vi "twitterSkipRemainingPhases.vi"(8 "error in":errorcluster, 9 "Prev Exp":T1(ring)=enum."Single Manip Jump", 10 "cell stats":T2={"Ihold (pA)"=-1000.0, "Rm (MOhms)"=0.0, "Ra (MOhms)"=0.0, "Cm (pF)"=0.0, "tau (ms)"=0.0, "Rt (MOhms)"=30.0, "Variance"=0.0, "STD"=0.0} {"STD" format="%010.2f"; "Variance" format="%010.2f"; "Rt (MOhms)" format="%010.2f"; "tau (ms)" format="%08.2g"; "Cm (pF)" format="%08.2f"; "Ra (MOhms)" format="%010.2f"; "Rm (MOhms)" format="%010.2f"; "Ihold (pA)" format="%010.2f"}, 11 "Prev Phase":string="B") -> (0 "error out":errorcluster, 2 "Skip Remaining":bool)   [LabVIEW 2019]
uses:
  <vilib>/LVH/i3 Twitter/Controls/Tweet.ctl
  wc_protocol_v1.003 Folder/whole_cell_protocol/Controls/cell_stats-v02.ctl
  <vilib>/LVH/i3 Twitter/i3-twitter.lvlib
panel:
  out "tweet sent":string
  in  "Continue Button":bool
  in  "Terminate Button":bool
  out "light on":bool
  out "New Tweets Read":T3[](array[typedef])
  # "The Cell/Patch looks to be comprimised, respond via twitter or the panel to proceed"
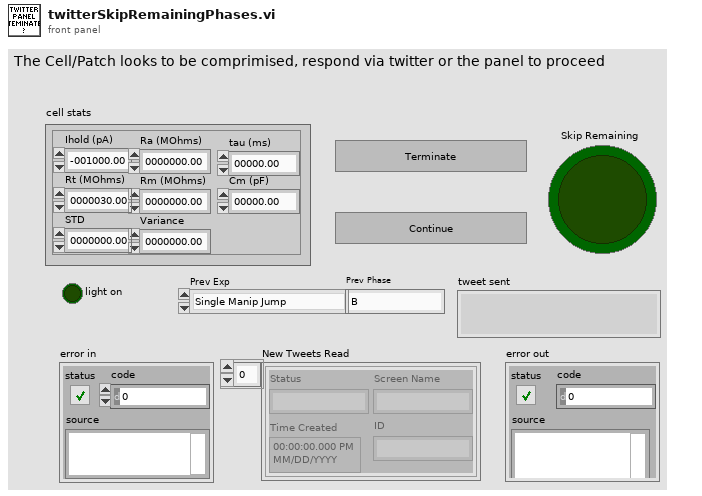
[diagram p1: front panel]
types:
  T1 = enum32{"Single Jump", "Solution Change", "Voltage Step", "Voltage Ramp", "Voltage Pulse", "Jump Train", "Paired Pulse", "Single Manip Jump", "Gap Free", "Multi M. Jump", "Current Pulse", "Current Ramp", "Gap Free Iclamp"}
  T2 = typedef "cell_stats-v02.ctl" = cluster{"Ihold (pA)":dbl, "Rm (MOhms)":dbl, "Ra (MOhms)":dbl, "Cm (pF)":dbl, "tau (ms)":dbl, "Rt (MOhms)":dbl, "Variance":dbl, "STD":dbl}
  T3 = typedef "i3-twitter.lvlib/Tweet.ctl" = cluster{"Status":string, "Time Created":timestamp, "Screen Name":string, "ID":string}
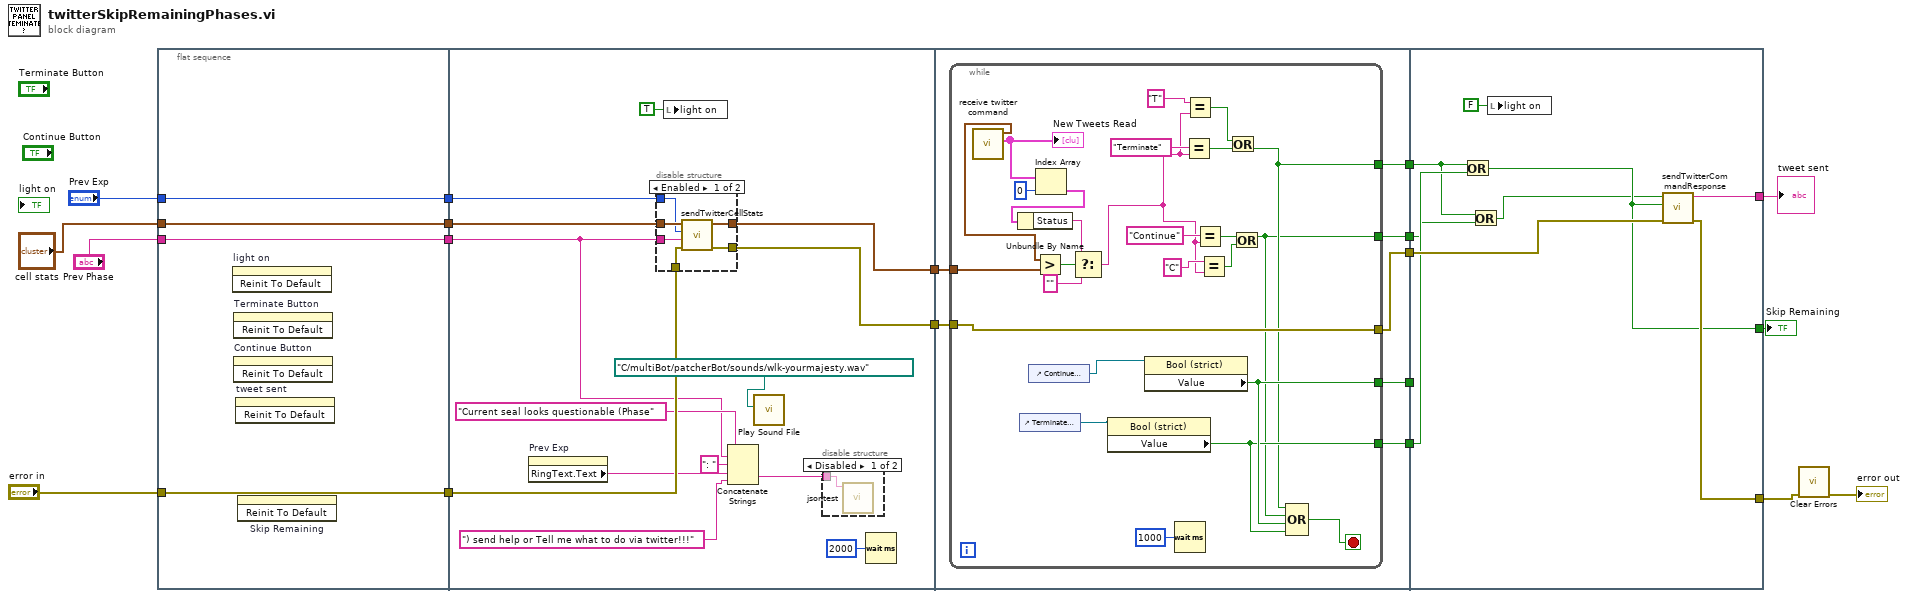
[diagram p0: block diagram]
diagram:
  n1 = flat-sequence {
    tunnel: "Prev Phase" -> [w20]
    tunnel: "Prev Exp" -> [w21]
    tunnel: "cell stats" -> [w22]
    tunnel: "error in" -> [w23]
    tunnel: [w23] -> w5
    tunnel: [w22] -> w4
    tunnel: [w21] -> w3
    tunnel: [w20] -> w2
    tunnel: [w35] -> w18
    tunnel: [w32] -> w7
    tunnel: w5 -> [w36]
    tunnel: w4 -> [w34]
    tunnel: w3 -> [w33]
    tunnel: w2 -> [w26]
    tunnel: w18 -> [w51]
    tunnel: [w50] -> w17
    tunnel: [w49] -> w15
    tunnel: [w48] -> w14
    tunnel: [w47] -> w13
    tunnel: [w46] -> w12
    tunnel: w7 -> [w45]
    tunnel: [w82] -> w19
    tunnel: w17 -> [w85]
    tunnel: [w84] -> w16
    tunnel: w15 -> [w80]
    tunnel: w14 -> [w81]
    tunnel: w13 -> [_]
    tunnel: w12 -> [w83]
    tunnel: [w78] -> w8
    frame #0 {
      n2 = invoke on="light on" class="Bool (strict)" method="Reinit To Default"() -> ()  [unwired: 3 in, 3 out]
      n3 = invoke on="Terminate Button" class="Bool (strict)" method="Reinit To Default"() -> ()  [unwired: 3 in, 3 out]
      n4 = invoke on="Continue Button" class="Bool (strict)" method="Reinit To Default"() -> ()  [unwired: 3 in, 3 out]
      n5 = invoke on="tweet sent" class="Str" method="Reinit To Default"() -> ()  [unwired: 3 in, 3 out]
      n6 = invoke on="Skip Remaining" class="Bool (strict)" method="Reinit To Default"() -> ()  [unwired: 3 in, 3 out]
    }
    frame #1 {
      n7 = property on="Prev Exp" class="Enum (strict)"() -> ("RingText.Text"=w25:string)  [unwired: 2 in, 2 out]
      n8 = disable-structure shown="Enabled" {
        disable-tunnel: w36 -> [w44 _]
        disable-tunnel: [w43 _] -> w35
        disable-tunnel: w34 -> [w42 _]
        disable-tunnel: w33 -> [w41 _]
        disable-tunnel: [w40 _] -> w32
        disable-tunnel: w26 -> [w39 _]
        frame Enabled {
          n9 = call "sendTwitterCellStats.vi"("error in"=w44, "Prev Phase"=w39, "Prev Exp"=w41, "cell stats"=w42) -> ("error out"=w43:errorcluster, "check Time"=w40:timestamp)  [unwired: 6 in]
        }
        frame Disabled {
        }
      }
      n10 = local write "light on"(TRUE ("light on")) -> ()
      n11 = Concatenate Strings("Current seal looks questionable (Phase" ("string"), w26, ": " ("string"), w25, ") send help or Tell me what to do via twitter!!!" ("string")) -> (w28:string)
      n12 = call <vilib>:"Play Sound File.vi"("path"=path "C:/multiBot/patcherBot/sounds/wlk-yourmajesty.wav") -> ()  [unwired: 9 in, 2 out]
      n13 = disable-structure shown="Disabled" {
        disable-tunnel: w28 -> [w38 _]
        frame Disabled {
          n14 = call "jsontest.vi"("string"=w38) -> ()  [unwired: 10 in, 1 out]
        }
        frame Enabled {
        }
      }
      n15 = Wait (ms)(milliseconds to wait=u32 2000) -> ()  [unwired: 1 out]
    }
    frame #2 {
      n16 = while {
        tunnel: w51 -> [w75]
        tunnel: [w75] -> w50
        tunnel: [w62] -> w49
        tunnel: [w61] -> w48
        tunnel: [w66] -> w47
        tunnel: [w65] -> w46
        tunnel: w45 -> [w54]
        stop <- w77 stop-if-true
        n17 = call "receive twitter command.vi"() -> ("New Tweets Read"=w71:T3[], "Time Stamp of Oldest Tweet"=w55:timestamp)  [unwired: 9 in, 1 out]
        "New Tweets Read" <- w71
        n18 = control-ref of="Terminate Button"() -> (w73:refnum<vi>)
        n19 = control-ref of="Continue Button"() -> (w74:refnum<vi>)
        n20 = Greater?(x=w55, y=w54) -> (0:w56:bool)
        n21 = Index Array(array=w71, index=0) -> (element=w58:T3)
        n22 = Unbundle By Name(w58) -> ("Status"=w57:string)
        n23 = Select(t=w57, s=w56, f="") -> (s? t:f=w53:string)
        n24 = property class="Bool (strict)"(reference=w73) -> ("Value"=w65:bool)  [unwired: 1 in, 2 out]
        n25 = property class="Bool (strict)"(reference=w74) -> ("Value"=w66:bool)  [unwired: 1 in, 2 out]
        n26 = Wait (ms)(milliseconds to wait=u32 1000) -> ()  [unwired: 1 out]
        n27 = Equal?(x="Terminate", y=w53) -> (x = y?=w68:bool)
        n28 = Equal?(x="T", y=w53) -> (x = y?=w59:bool)
        n29 = Equal?(x="Continue", y=w53) -> (x = y?=w67:bool)
        n30 = Equal?(x="C", y=w53) -> (x = y?=w60:bool)
        n31 = Or(x=w59, y=w68) -> (x .or. y?=w62:bool)
        n32 = Or(x=w67, y=w60) -> (x .or. y?=w61:bool)
        n33 = Compound Arithmetic op=OR(w62, w61, w66, w65) -> (w77:bool)
      }
    }
    frame #3 {
      n34 = Or(x=w80, y=w83) -> (x .or. y?=w82:bool)
      n35 = Or(x=w80, y=w81) -> (x .or. y?=w79:bool)
      n36 = local write "light on"(FALSE ("light on")) -> ()
      n37 = call "sendTwitterCommandResponse.vi"("error in"=w85, "TeminateOrContinue"=w82, "TwitterOrPanel"=w79) -> ("error out"=w84:errorcluster, "tweet sent"=w78:string)  [unwired: 7 in]
    }
  }
  n38 = call <vilib>:"Clear Errors.vi"("error in (no error)"=w16) -> ("error out"=→"error out":errorcluster)  [unwired: 5 in, 1 out]
  "Skip Remaining" <- w19
  "tweet sent" <- w8
